vi "VLW_Phi.vi"(11 "VL/W":dbl[](array[numeric])) -> (2 "PhiL":dbl, 3 "PhiR":dbl)   [LabVIEW 2011]
uses:
  <vilib>/Analysis/baseanly.llb/Real Inverse Matrix.vi
  <vilib>/Analysis/Matrix/Numeric/Conversions/Array To Matrix - RA.vi
  <vilib>/Analysis/baseanly.llb/Real A x B.vi
  <vilib>/Analysis/NI_AALBase.lvlib
  <vilib>/Analysis/Matrix/NI_Matrix.lvlib
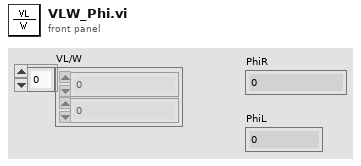
[diagram p1: front panel]
types:
  T1 = typedef "NI_Matrix.lvlib/RealMatrix.ctl" = dbl[][]
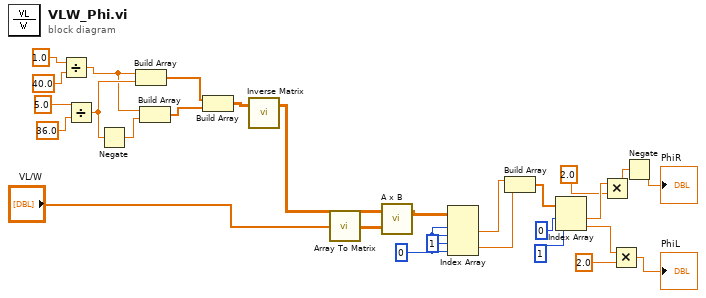
[diagram p0: block diagram]
diagram:
  w5 = 0 ("index (col)")
  n1 = Divide(x=1.0, y=40.0) -> (x/y=w22:dbl)
  n2 = Divide(x=5.0, y=36.0) -> (x/y=w24:dbl)
  n3 = Negate(x=w24) -> (-x=w23:dbl)
  n4 = Build Array(w22, w24) -> (w26:dbl[])
  n5 = Build Array(w22, w23) -> (w25:dbl[])
  n6 = Build Array(w26, w25) -> (w17:T1)
  n7 = call-poly <vilib>:"Inverse Matrix.vi"("Input Matrix"=w17) -> ("Inverse Matrix"=w2:T1)  [unwired: 1 in, 1 out]
  n8 = call-poly <vilib>:"Array To Matrix.vi"("Real 1D Array"="VL/W") -> ("Real Matrix (Column Vector)"=w3:T1)
  n9 = call-poly <vilib>:"A x B.vi"("B"=w3, "A"=w2) -> ("A x B"=w1:T1)  [unwired: 1 out]
  n10 = Index Array(array=w1, index (row) #1=w5, index (col) #1=w5, index (row) #2=1 ("index (row)"), index (col) #2=w5) -> (element #1=w8:dbl, element #2=w7:dbl)
  n11 = Build Array(w8, w7) -> (w6:dbl[])
  n12 = Index Array(array=w6, index #1=0 ("index"), index #2=1 ("index")) -> (element #1=w15:dbl, element #2=w14:dbl)
  n13 = Multiply(x=w15, y=2.0) -> (x*y=w10:dbl)
  n14 = Multiply(x=w14, y=2.0) -> (x*y=→"PhiL":dbl)
  n15 = Negate(x=w10) -> (-x=→"PhiR":dbl)
